vi "rad7v1.1.vi"() -> ()   [LabVIEW 2012]
uses:
  <vilib>/Platform/TimedLoop/XDataNode/timing_clust.ctl
  <vilib>/Platform/TimedLoop/XDataNode/nitl_modes.ctl
  <vilib>/Platform/TimedLoop/XDataNode/wakeup.ctl
  <vilib>/Instr/_visa.llb/VISA Configure Serial Port (Instr).vi
  <vilib>/Platform/TimedLoop/XDataNode/XDataNode.xnode
  <vilib>/Platform/TimedLoop/XDataNode/XDNodeRunTimeDep.lvlib
panel:
  in  "Timestamp":bool
  out "Numeric 2":i32
  in  "Path":path=path "C:/Users/reuterc/Documents/GitHub/modudaq/rad7data.txt"
  in  "VISA resource name":refnum<visa-resource-name>
  out "Numeric":i32
  in  "Loop Time (s)":dbl=1.0
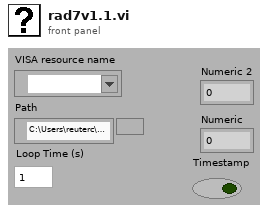
[diagram p1: front panel]
types:
  T1 = typedef "XDNodeRunTimeDep.lvlib/timing_clust.ctl" = cluster{"Expected End [f-1]":u64, "Actual End [f-1]":u64, "Finished Late? [f-1]":bool, "Expected End [i-1]":u64, "Actual End [i-1]":u64, "Finished Late? [i-1]":bool, "Expected Start [i]":u64, "Actual Start [i]":u64, "Expected Start [f]":u64, "Actual Start [f]":u64, "Source Name":string, "Structure Name":string, "Period":i64, "Deadline":i64, "Offset":i64, "Start":i64, "Priority":i32, "Timeout":i32, "Mode":T2, "Wakeup Reason":T3, "Error":errorcluster, "Source Type":string, "Secondary Source Type":string, "Global End Time":u64, "Global Start Time":u64, "Frame Duration":u64, "Iteration Duration":u64, "Assigned CPU":i32, "I/O Scan Engine Mode":u32}
  T2 = typedef "XDNodeRunTimeDep.lvlib/nitl_modes.ctl" = enum32{"No Change", "Process missed periods, maintain original phase", "Discard missed periods, maintain original phase", "Process missed periods, ignore original phase", "Discard missed periods, ignore original phase"}
  T3 = typedef "XDNodeRunTimeDep.lvlib/wakeup.ctl" = enum32{"Normal", "Aborted", "Asynchronous wakeup", "Timing source error", "Timed loop error", "Timeout"}
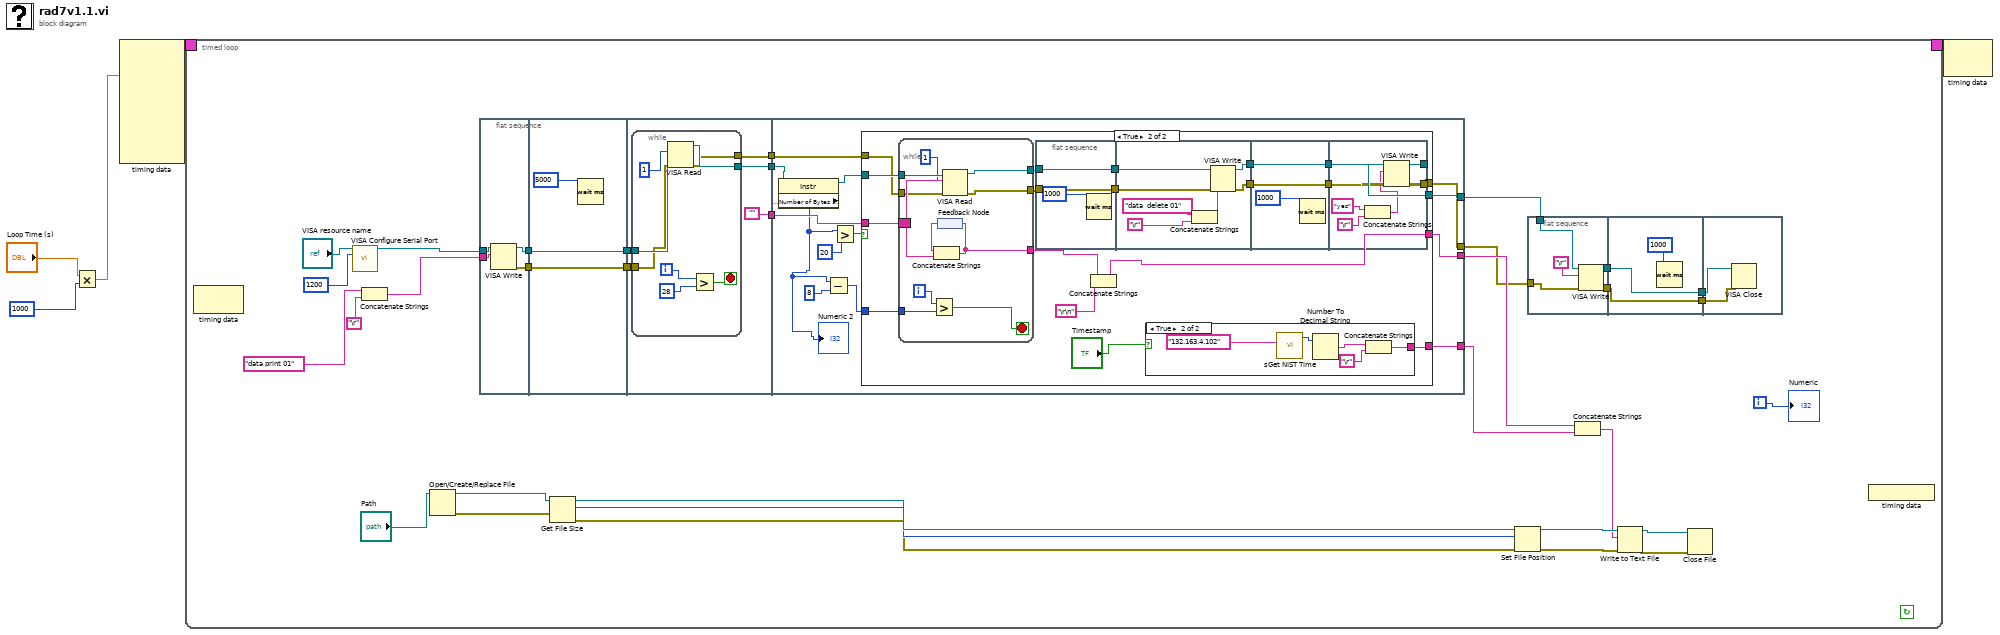
[diagram p0: block diagram]
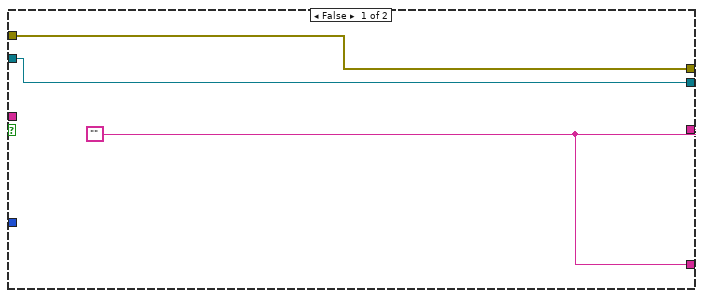
[diagram p2: hidden frame]
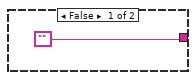
[diagram p3: hidden frame]
diagram:
  n1 = Multiply(x="Loop Time (s)", y=1000) -> (x*y=w1:dbl)
  n2 = node-c288(w1) -> (w5:T1)  [unwired: 7 in]
  n3 = timed-loop {
    timing: w5 -> [_]
    timing-out: [_] -> w4
    i -> [w6]
    stop <- _ continue-if-true
    n4 = node-c288() -> ()  [unwired: 1 in, 1 out]
    n5 = call-poly "VISA Configure Serial Port"("VISA resource name"="VISA resource name", "baud rate (9600)"=1200) -> ("VISA resource name out"=w21:refnum<visa-resource-name>)  [unwired: 12 in, 1 out]
    n6 = Concatenate Strings("data print 01" ("Command"), "\r") -> (w20:string)
    n7 = Open/Create/Replace File(file path (use dialog)="Path") -> (refnum out=w37:refnum<file>, error out=w36:errorcluster)  [unwired: 5 in, 1 out]
    n8 = flat-sequence {
      tunnel: w20 -> [w52]
      tunnel: w21 -> [w51]
      tunnel: [w50] -> w19
      tunnel: [w49] -> w17
      tunnel: w19 -> [w55]
      tunnel: [w55] -> w18
      tunnel: w17 -> [w54]
      tunnel: [w54] -> w16
      tunnel: [w60] -> w24
      tunnel: [""] -> w23
      tunnel: [w58] -> w22
      tunnel: w18 -> [w57]
      tunnel: w16 -> [w56]
      tunnel: [w81] -> w11
      tunnel: w24 -> [w79]
      tunnel: w23 -> [w80]
      tunnel: [w73] -> w13
      tunnel: w22 -> [w75]
      tunnel: [w74] -> w12
      tunnel: [w70] -> w14
      frame #0 {
        n9 = VISA Write(VISA resource name=w51, write buffer=w52) -> (VISA resource name out=w50:refnum<visa-resource-name>, error out=w49:errorcluster)  [unwired: 1 in, 1 out]
      }
      frame #1 {
        n10 = Wait (ms)(milliseconds to wait=5000) -> ()  [unwired: 1 out]
      }
      frame #2 {
        n11 = while {
          tunnel: w57 -> [w67]
          tunnel: [w63] -> w60
          tunnel: w56 -> [w62]
          tunnel: [w61] -> w58
          i -> [w66]
          stop <- w64 stop-if-true
          n12 = VISA Read(VISA resource name=w67, byte count=1, error in (no error)=w62) -> (VISA resource name out=w63:refnum<visa-resource-name>, error out=w61:errorcluster)  [unwired: 2 out]
          n13 = Greater?(x=w66, y=28) -> (0:w64:bool)
        }
      }
      frame #3 {
        n14 = property class="Instr"(reference=w79) -> (reference out=w78:refnum<visa-resource-name>, "Serial Settings:Number of Bytes at Serial Port"=w69:u32)  [unwired: 1 in, 1 out]
        "Numeric 2" <- w69
        n15 = Subtract(x=w69, y=8) -> (x-y=w71:u32)
        n16 = Greater?(x=w69, y=20) -> (0:w77:bool)
        n17 = case shown="True" w77 {
          tunnel: [w84 w97] -> w81
          tunnel: w80 -> [_ w103]
          tunnel: [w82 w89] -> w73
          tunnel: w78 -> [w84 w102]
          tunnel: w71 -> [_ w101]
          tunnel: w75 -> [w83 w96]
          tunnel: [w83 w94] -> w74
          tunnel: [w82 w86] -> w70
          frame False {
            w82 = ""
          }
          frame True {
            n18 = while {
              tunnel: w102 -> [w136]
              border: w103 -> [_]
              tunnel: [w137] -> w99
              tunnel: w101 -> [w134]
              tunnel: [w132] -> w98
              tunnel: w96 -> [w131]
              tunnel: [w130] -> w95
              i -> [w138]
              stop <- w133 stop-if-true
              n19 = Greater?(x=w138, y=w134) -> (0:w133:bool)
              n20 = feedback #1() -> (w139:string)
              n21 = VISA Read(VISA resource name=w136, byte count=1, error in (no error)=w131) -> (VISA resource name out=w132:refnum<visa-resource-name>, read buffer=w140:string, error out=w130:errorcluster)  [unwired: 1 out]
              n22 = Concatenate Strings(w139, w140) -> (w137:string)
              n23 = feedback-in #1(w137) -> ()
            }
            n24 = flat-sequence {
              tunnel: w95 -> [w111]
              tunnel: w98 -> [w112]
              tunnel: [w112] -> w88
              tunnel: [w111] -> w87
              tunnel: [w116] -> w93
              tunnel: [w113] -> w91
              tunnel: w88 -> [w115]
              tunnel: w87 -> [w114]
              tunnel: w93 -> [w122]
              tunnel: [w122] -> w92
              tunnel: w91 -> [w121]
              tunnel: [w121] -> w90
              tunnel: w92 -> [w126]
              tunnel: [w125] -> w97
              tunnel: w90 -> [w124]
              tunnel: [w123] -> w94
              frame #0 {
                n25 = Wait (ms)(milliseconds to wait=1000) -> ()  [unwired: 1 out]
              }
              frame #1 {
                n26 = Concatenate Strings("data  delete 01", "\r") -> (w117:string)
                n27 = VISA Write(VISA resource name=w115, write buffer=w117, error in (no error)=w114) -> (VISA resource name out=w116:refnum<visa-resource-name>, error out=w113:errorcluster)  [unwired: 1 out]
              }
              frame #2 {
                n28 = Wait (ms)(milliseconds to wait=1000) -> ()  [unwired: 1 out]
              }
              frame #3 {
                n29 = Concatenate Strings("yes", "\r") -> (w127:string)
                n30 = VISA Write(VISA resource name=w126, write buffer=w127, error in (no error)=w124) -> (VISA resource name out=w125:refnum<visa-resource-name>, error out=w123:errorcluster)  [unwired: 1 out]
              }
            }
            n31 = Concatenate Strings(w99, "\r\n") -> (w89:string)
            n32 = case shown="True" "Timestamp" {
              tunnel: ["" w105] -> w86
              frame False {
              }
              frame True {
                n33 = call "sGet NIST Time.vi"("IP Address of NIST Server"="132.163.4.102") -> ("NTP Time"=w108:u64)  [unwired: 1 in, 2 out]
                n34 = Number To Decimal String(number=w108) -> (decimal integer string=w106:string)  [unwired: 1 in]
                n35 = Concatenate Strings(w106, "\r") -> (w105:string)
              }
            }
          }
        }
      }
    }
    n36 = Get File Size(file=w37, error in=w36) -> (refnum out=w29:refnum<file>, size (in bytes)=w27:i64, 0:w26:errorcluster)
    n37 = Set File Position(offset (in bytes) (0)=w27, refnum=w29, error in=w26) -> (refnum out=w28:refnum<file>, error out=w25:errorcluster)  [unwired: 1 in]
    n38 = flat-sequence {
      tunnel: w12 -> [w42]
      tunnel: w11 -> [w41]
      tunnel: [w40] -> w9
      tunnel: [w39] -> w7
      tunnel: [w45] -> w10
      tunnel: w9 -> [w45]
      tunnel: [w44] -> w8
      tunnel: w7 -> [w44]
      tunnel: w10 -> [w48]
      tunnel: w8 -> [w47]
      frame #0 {
        n39 = VISA Write(VISA resource name=w41, write buffer="\r", error in (no error)=w42) -> (VISA resource name out=w40:refnum<visa-resource-name>, error out=w39:errorcluster)  [unwired: 1 out]
      }
      frame #1 {
        n40 = Wait (ms)(milliseconds to wait=1000) -> ()  [unwired: 1 out]
      }
      frame #2 {
        n41 = VISA Close(VISA resource name=w48, error in (no error)=w47) -> ()  [unwired: 1 out]
      }
    }
    n42 = Concatenate Strings(w13, w14) -> (w15:string)
    n43 = Write to Text File(file (use dialog)=w28, text=w15, error in=w25) -> (refnum out=w35:refnum<file>, error out=w34:errorcluster)  [unwired: 1 in, 1 out]
    n44 = Close File(refnum=w35, error in=w34) -> ()  [unwired: 2 out]
    n45 = node-c288() -> ()  [unwired: 1 out]
    "Numeric" <- w6
  }
  n46 = node-c288(w4) -> ()  [unwired: 1 out]
